vi "StringToEightByteReal.vi"(8 "error in (no error)":errorcluster, 11 "String":string) -> (0 "error out":errorcluster, 3 "Array":dbl[](array[numeric]))   [LabVIEW 2019]
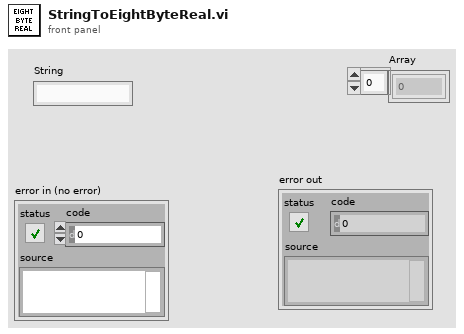
[diagram p1: front panel]
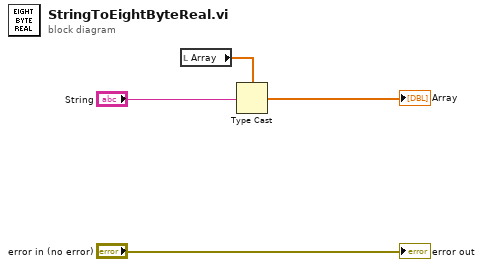
[diagram p0: block diagram]
diagram:
  n1 = local read "Array"() -> (w2:dbl[])
  n2 = Type Cast(type=w2, x="String") -> (*(type *) &x=→"Array":dbl[])
  "error out" <- "error in (no error)"
